vi "PC_DPG to DECM.vi"() -> ()   [LabVIEW 2021]
uses:
  Digital Edge Count Measurement/Typedefs/Measurement Settings.ctl
  Digital Edge Count Measurement/Typedefs/Wait Type.ctl
  Digital Edge Count Measurement/Typedefs/Timer - Trigger Settings.ctl
  Digital Pulse Generation/Typedefs/Digital Pulse Settings.ctl
  Digital Pulse Generation/Typedefs/Actual Pulse Settings.ctl
  Common/Typedefs/Execution Options - Measure.ctl
  Digital Edge Count Measurement/DAQ_Digital Edge Count Measurement.lvlib
  Digital Pulse Generation/DAQ_Digital Pulse Generation.lvlib
panel:
  out "error out":errorcluster
  out "Edge Counts":u32=5
  out "Actual Pulse Settings":T1={"High Time (s)"=0.0005, "Low Time (s)"=0.0005, "Generation Time (s)"=0.005} {"Low Time (s)" format="%.2p"; "High Time (s)" format="%.2p"; "Generation Time (s)" format="%.2p"}
  in  "Digital Pulse Settings":T2={"High Time (s)"=0.0005, "Low Time (s)"=0.0005, "Number of Pulses"=5} {"Low Time (s)" format="%.2p"; "High Time (s)" format="%.2p"}
  in  "Timer - Trigger Settings":T3={"Trigger Type"=enum."Digital Start", "Digital Start Trigger Source"="/Dev1/PFI3", "Digital Start Trigger Edge"=10280} {"Digital Start Trigger Edge" items=["Rising"=10280, "Falling"=10171]}
  in  "Counter Settings":T4={"Active Edge"=10171, "Duration (s)"=0.005, "Wait Type"=enum."Hardware Timed"} {"Duration (s)" format="%.2p"; "Active Edge" items=["Rising"=10280, "Falling"=10171]}
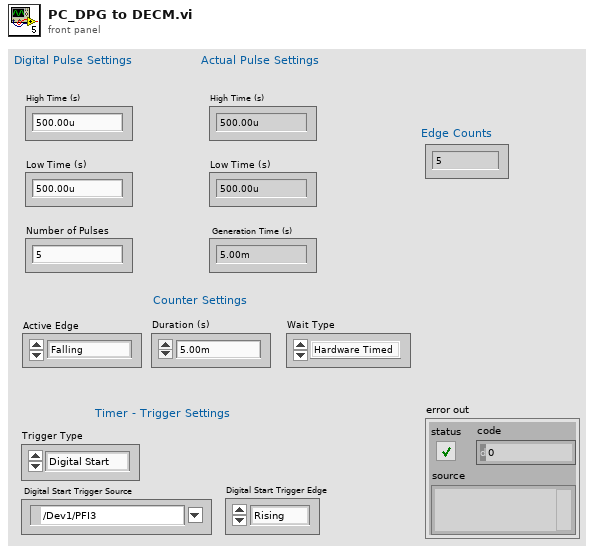
[diagram p1: front panel]
types:
  T1 = typedef "DAQ_Digital Pulse Generation.lvlib/Actual Pulse Settings.ctl" = cluster{"High Time (s)":dbl, "Low Time (s)":dbl, "Generation Time (s)":dbl}
  T2 = typedef "DAQ_Digital Pulse Generation.lvlib/Digital Pulse Settings.ctl" = cluster{"High Time (s)":dbl, "Low Time (s)":dbl, "Number of Pulses":i32}
  T3 = typedef "DAQ_Digital Edge Count Measurement.lvlib/Timer - Trigger Settings.ctl" = cluster{"Trigger Type":enum16{"No Trigger", "Digital Start"}, "Digital Start Trigger Source":tag, "Digital Start Trigger Edge":i32}
  T4 = typedef "DAQ_Digital Edge Count Measurement.lvlib/Measurement Settings.ctl" = cluster{"Active Edge":i32, "Duration (s)":dbl, "Wait Type":T5}
  T5 = typedef "DAQ_Digital Edge Count Measurement.lvlib/Wait Type.ctl" = enum16{"Hardware Timed", "Software Timed"}
  T6 = typedef "Execution Options - Measure.ctl" = enum16{"Configure & Measure", "Configure only", "Measure only"}
  T7 = typedef "DAQ_Digital Edge Count Measurement.lvlib/DAQmx Tasks.ctl" = cluster{"Counter DAQmx Task":refnum<k21>, "Timer DAQmx Task":refnum<k21>}
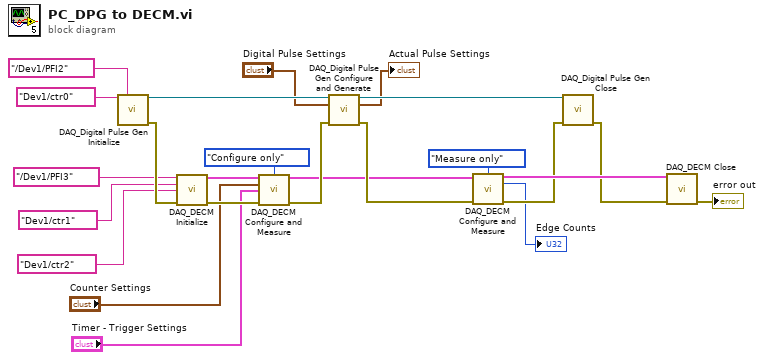
[diagram p0: block diagram]
diagram:
  n1 = call "DAQ_Digital Pulse Gen Initialize.vi"("Physical Channel (Counter)"=tag "Dev1/ctr0", "Output Terminal"=tag "/Dev1/PFI2") -> ("DAQmx Task Out"=w22:refnum<k21>, "error out"=w20:errorcluster)  [unwired: 12 in]
  n2 = call "DAQ_DECM Initialize.vi"("Input Terminal"=tag "/Dev1/PFI3", "Counter - Edge Counting"=tag "Dev1/ctr1", "Counter - Timer"=tag "Dev1/ctr2", "error in"=w20) -> ("DAQmx Tasks"=w16:T7, "error out"=w15:errorcluster)  [unwired: 10 in]
  n3 = call "DAQ_DECM Configure and Measure.vi"("DAQmx Tasks In"=w16, "Execution Option"=Execution_Options_-_Measure."Configure only", "Counter Settings"="Counter Settings", "Timer - Trigger Settings"="Timer - Trigger Settings", "error in"=w15) -> ("DAQmx Tasks Out"=w10:T7, "error out"=w12:errorcluster)  [unwired: 8 in, 1 out]
  n4 = call "DAQ_Digital Pulse Gen Configure and Generate.vi"("DAQmx Task In"=w22, "Digital Pulse Settings"="Digital Pulse Settings", "error in"=w12) -> ("DAQmx Task Out"=w21:refnum<k21>, "Actual Pulse Settings"=→"Actual Pulse Settings":T1, "error out"=w11:errorcluster)  [unwired: 10 in]
  n5 = call "DAQ_DECM Configure and Measure.vi"("DAQmx Tasks In"=w10, "Execution Option"=Execution_Options_-_Measure."Measure only", "error in"=w11) -> ("DAQmx Tasks Out"=w9:T7, "Edge Counts"=→"Edge Counts":u32, "error out"=w8:errorcluster)  [unwired: 10 in]
  n6 = call "DAQ_Digital Pulse Gen Close.vi"("DAQmx Task In"=w21, "error in"=w8) -> ("error out"=w7:errorcluster)  [unwired: 13 in]
  n7 = call "DAQ_DECM Close.vi"("DAQmx Tasks"=w9, "error in"=w7) -> ("error out"=→"error out":errorcluster)  [unwired: 13 in]
